vi "example_01_single_plot.vi"() -> ()   [LabVIEW 2015, in "lv-graph-global.lvlib"]
uses:
  lv-graph-global.lvlib
  _controls/configuration.ctl
  _controls/store_method.ctl
  advanced/write-point.vi
  advanced/read-data.vi
  <userlib>/antonio-alexander/lv-graph/public/advanced/build_graph-single_axis.vi
  <userlib>/antonio-alexander/lv-graph/lv-graph.lvlib
panel:
  in  "clear":bool
  out "single_x_axis":T1(graph)
  in  "realtime":bool=TRUE
  in  "data_rate_ms":u32=10
  in  "refresh_rate_ms":u32=250
  in  "configuration":T2={"store_method"=enum."fixed", "rows"=1000, "columns"=2}
  in  "stop":bool
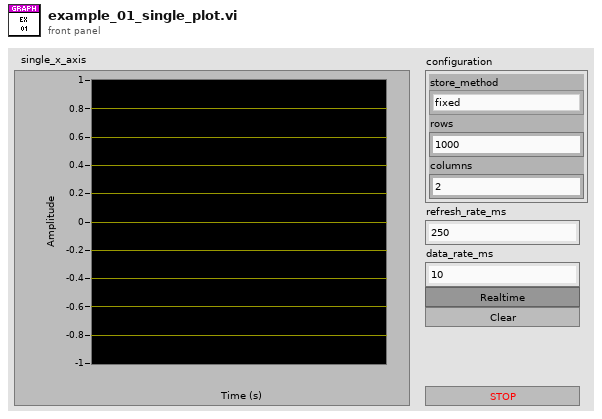
[diagram p1: front panel]
types:
  T1 = cluster{"Time [] out":dbl[], "Data[][] out":dbl[]}[]
  T2 = typedef "lv-graph-global.lvlib/configuration.ctl" = cluster{"store_method":T3, "rows":i32, "columns":i32}
  T3 = typedef "lv-graph-global.lvlib/store_method.ctl" = enum16{"<store_method>", "fixed", "grow"}
  T4 = enum8{"Enabled", "Disabled", "Disabled and Grayed Out"}
  T5 = cluster{"x_scale_maximum":dbl, "x_scale_minimum":dbl, "y_scale_maximum":dbl, "y_scale_minimum":dbl}
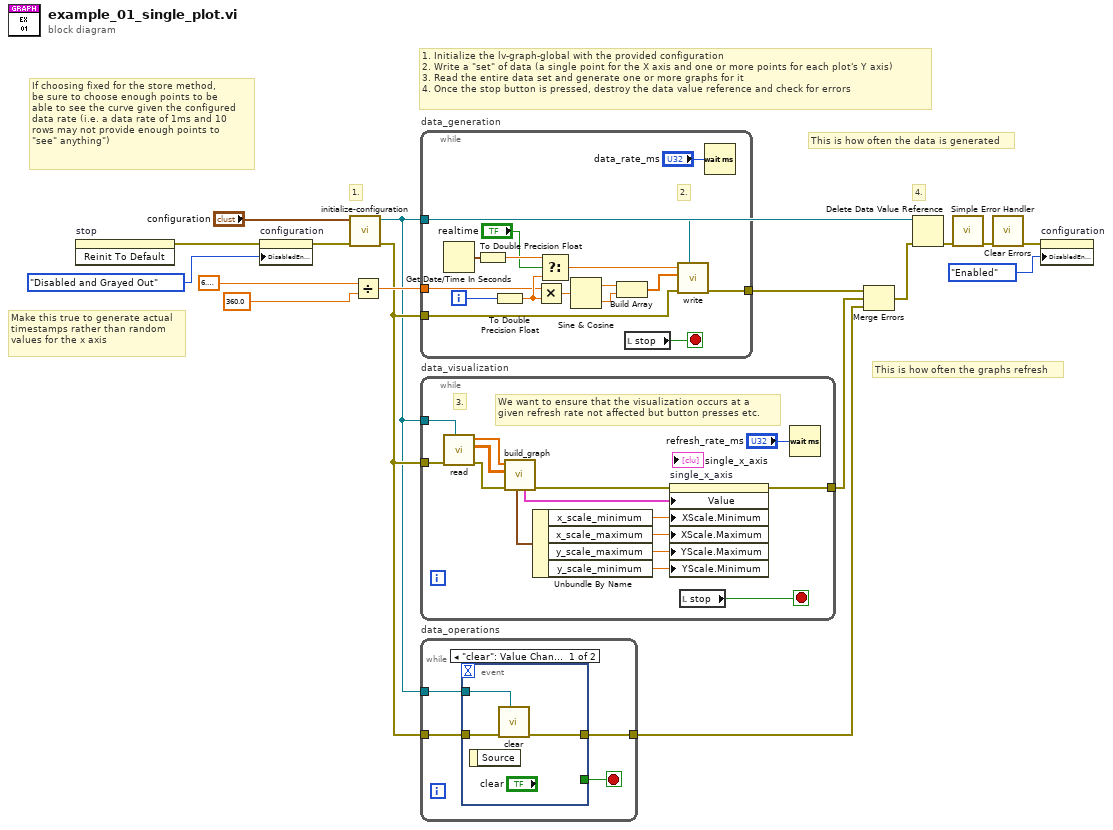
[diagram p0: block diagram]
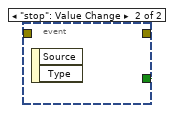
[diagram p2: hidden frame]
diagram:
  # "Make this true to generate actual\ntimestamps rather than random \nvalues for the x axis"
  # "This is how often the data is generated"
  # "This is how often the graphs refresh"
  # "If choosing fixed for the store method,\nbe sure to choose enough points to be\nable to see the curve given the configured\ndata rate (i.e. a data rate of 1ms and 10\nrows may not provide enough points to\n\"see\" anything\")"
  # "1. Initialize the lv-graph-global with the provided configuration\n2. Write a \"set\" of data (a single point for the X axis and one or more points for each plot's Y axis)\n3. Read the entire data set and generate one or more graphs for it\n4. Once the stop button is pressed, destroy the data value reference and check for errors"
  # "4."
  # "1."
  n1 = invoke on="stop" class="Bool (strict)" method="Reinit To Default"() -> (error out=w6:errorcluster)  [unwired: 3 in, 2 out]
  n2 = property on="configuration" class="Clust (strict)"(error in=w6, "DisabledEnum"=T4."Disabled and Grayed Out" ("Disabled")) -> (error out=w5:errorcluster)  [unwired: 1 in, 1 out]
  n3 = call "initialize-configuration.vi"("error in (no error)"=w5, "configuration"="configuration") -> ("error out"=w10:errorcluster, "dvr"=w9:refnum<data-value>)  [unwired: 8 in]
  n4 = Divide(x=6.283185307179586, y=360.0) -> (x/y=w12:dbl)
  n5 = while "data_generation" {
    tunnel: w10 -> [w24]
    tunnel: [w23] -> w17
    tunnel: w9 -> [w20]
    tunnel: w12 -> [w19]
    i -> [w31]
    stop <- w32 stop-if-true
    # "2."
    n6 = Get Date/Time In Seconds() -> (seconds since 1Jan1904=w33:timestamp)
    n7 = To Double Precision Float(number=w33) -> (double precision float=w29:dbl)
    n8 = To Double Precision Float(number=w31) -> (double precision float=w28:dbl)
    n9 = Multiply(x=w19, y=w28) -> (x*y=w27:dbl)
    n10 = Select(t=w29, s="realtime", f=w28) -> (s? t:f=w22:dbl)
    n11 = Sine & Cosine(0:w27) -> (1:w26:dbl, 2:w25:dbl)
    n12 = Build Array(w26, w25) -> (w21:dbl[])
    n13 = local read "stop"() -> (w32:bool)
    n14 = call-poly "write.vi"("dvr"=w20, "error in (no error)"=w24, "y_axis"=w21, "x_axis"=w22) -> ("error out"=w23:errorcluster)  [unwired: 6 in, 1 out]
    n15 = Wait (ms)(milliseconds to wait="data_rate_ms") -> ()  [unwired: 1 out]
  }
  n16 = while "data_visualization" {
    tunnel: w10 -> [w47]
    tunnel: w9 -> [w36]
    tunnel: [w34] -> w7
    stop <- w35 stop-if-true
    # "We want to ensure that the visualization occurs at a\ngiven refresh rate not affected but button presses etc."
    # "3."
    n17 = call-poly "read.vi"("dvr"=w36, "error in (no error)"=w47) -> ("error out"=w41:errorcluster, "y_axis"=w37:dbl[][], "x_axis"=w40:dbl[])  [unwired: 6 in, 1 out]
    n18 = call-poly <userlib>:"build_graph.vi"("error in (no error)"=w41, "y_axis"=w37, "x_axis"=w40) -> ("error out"=w42:errorcluster, "graph_data"=w38:cluster{dbl[], dbl[]}[], "scale_ranges"=w39:T5)  [unwired: 6 in]
    n19 = Unbundle By Name(w39) -> ("x_scale_minimum"=w44:dbl, "x_scale_maximum"=w43:dbl, "y_scale_maximum"=w45:dbl, "y_scale_minimum"=w46:dbl)
    n20 = property on="single_x_axis" class="XYGraph (strict)"(error in=w42, "Value"=w38, "XScale.Minimum"=w44, "XScale.Maximum"=w43, "YScale.Maximum"=w45, "YScale.Minimum"=w46) -> (error out=w34:errorcluster)  [unwired: 1 in, 1 out]
    n21 = local read "stop"() -> (w35:bool)
    n22 = Wait (ms)(milliseconds to wait="refresh_rate_ms") -> ()  [unwired: 1 out]
  }
  n23 = while "data_operations" {
    tunnel: w10 -> [w52]
    tunnel: w9 -> [w51]
    tunnel: [w49] -> w8
    stop <- w50 stop-if-true
    n24 = event shown="[0] \"clear\": Value Change" {
      selector: _ -> [_ _]
      dyn-events: _ -> [_ _]
      timeout: _ -> [_ _]
      tunnel: w52 -> [w55 _]
      tunnel: w51 -> [w54 _]
      tunnel: [_ TRUE] -> w50
      tunnel: [w53 _] -> w49
      event "clear": Value Change {
        n25 = event-data() -> ()  [unwired: 1 in, 1 out]
        n26 = call "clear.vi"("dvr"=w54, "error in (no error)"=w55) -> ("error out"=w53:errorcluster)  [unwired: 9 in]
      }
      event "stop": Value Change {
        n27 = event-data() -> ()  [unwired: 1 in, 2 out]
      }
    }
  }
  n28 = Merge Errors(w17, w7, w8) -> (w15:errorcluster)
  n29 = Delete Data Value Reference(data value reference=w9, error in=w15) -> (error out=w11:errorcluster)  [unwired: 1 out]
  n30 = call <vilib>:"Simple Error Handler.vi"("error in (no error)"=w11) -> ("error out"=w4:errorcluster)  [unwired: 4 in, 4 out]
  n31 = call <vilib>:"Clear Errors.vi"("error in (no error)"=w4) -> ("error out"=w3:errorcluster)  [unwired: 5 in, 1 out]
  n32 = property on="configuration" class="Clust (strict)"(error in=w3, "DisabledEnum"=T4."Enabled" ("Disabled")) -> ()  [unwired: 1 in, 2 out]
